vi "Asynchronous - Update RT to BC and RT to RT Data.vi"(5 "Raw Values (RT to BC)":T4, 7 "Map (RT to BC)":T1[](array[typedef]) {"Word Data Reference" format="%.0x"}, 8 "Error (in)":errorcluster, 9 "Updated FIFO Index []":i32[](array[numeric]), 10 "U16 []":u16[](array[numeric])) -> (0 "Error (out)":errorcluster)   [LabVIEW 2019, in "Ballard MIL-1553 Engine.lvlib"]
uses:
  Ballard MIL-1553 Engine.lvlib
  Controls/RT Async_Raw Values.ctl
  Controls/RT Async_Raw Values to Messages Index_Association.ctl
  Controls/RT Async_Map RT2BC.ctl
  <vilib>/NI VeriStand/Custom Device API/Data Reference.ctl
  Controls/RT Async_Map_Type.ctl
  <userlib>/_OpenG.lib/array/array.llb/Remove Duplicates from 1D Array (I32)__ogtk.vi
  <instrlib>/BTI1553Lib/BTI1553LV.lvlib
  <vilib>/NI VeriStand/Custom Device Tools/Custom Device Utility Library/Custom Device Utility Library.lvlib
  <vilib>/NI VeriStand/Custom Device API/Custom Device API.lvlib
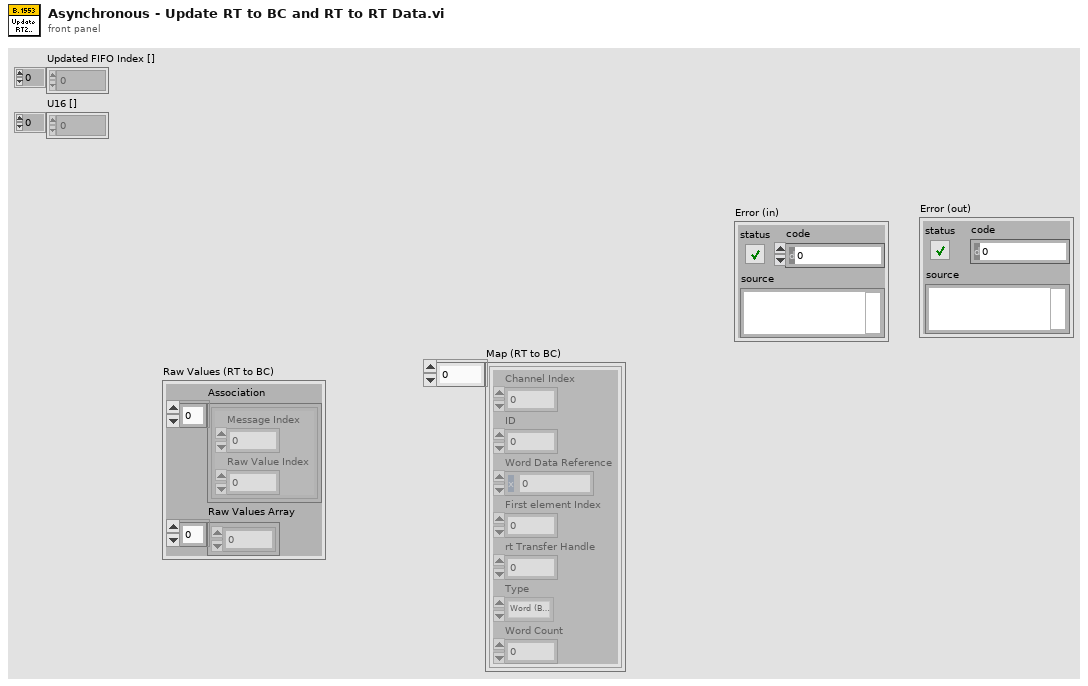
[diagram p1: front panel]
types:
  T1 = typedef "Ballard MIL-1553 Engine.lvlib/RT Async_Map RT2BC.ctl" = cluster{"Channel Index":i32, "ID":i32, "Word Data Reference":T2, "First element Index":i32, "rt Transfer Handle":u64, "Type":T3, "Word Count":i32}
  T2 = typedef "Custom Device API.lvlib/Data Reference.ctl" = i32
  T3 = typedef "Ballard MIL-1553 Engine.lvlib/RT Async_Map_Type.ctl" = enum16{"Word (BC to RT)", "Word (MC (Rx))", "Acyclic Message Trigger", "Word (RT to ..)", "Word (RT to RT)", "Word (MC (Tx))", "RT Status", "BC Commands", "RT Commands"}
  T4 = typedef "Ballard MIL-1553 Engine.lvlib/RT Async_Raw Values.ctl" = cluster{"Association":T5[], "Raw Values Array":u16[]}
  T5 = typedef "Ballard MIL-1553 Engine.lvlib/RT Async_Raw Values to Messages Index_Association.ctl" = cluster{"Message Index":i32, "Raw Value Index":i32}
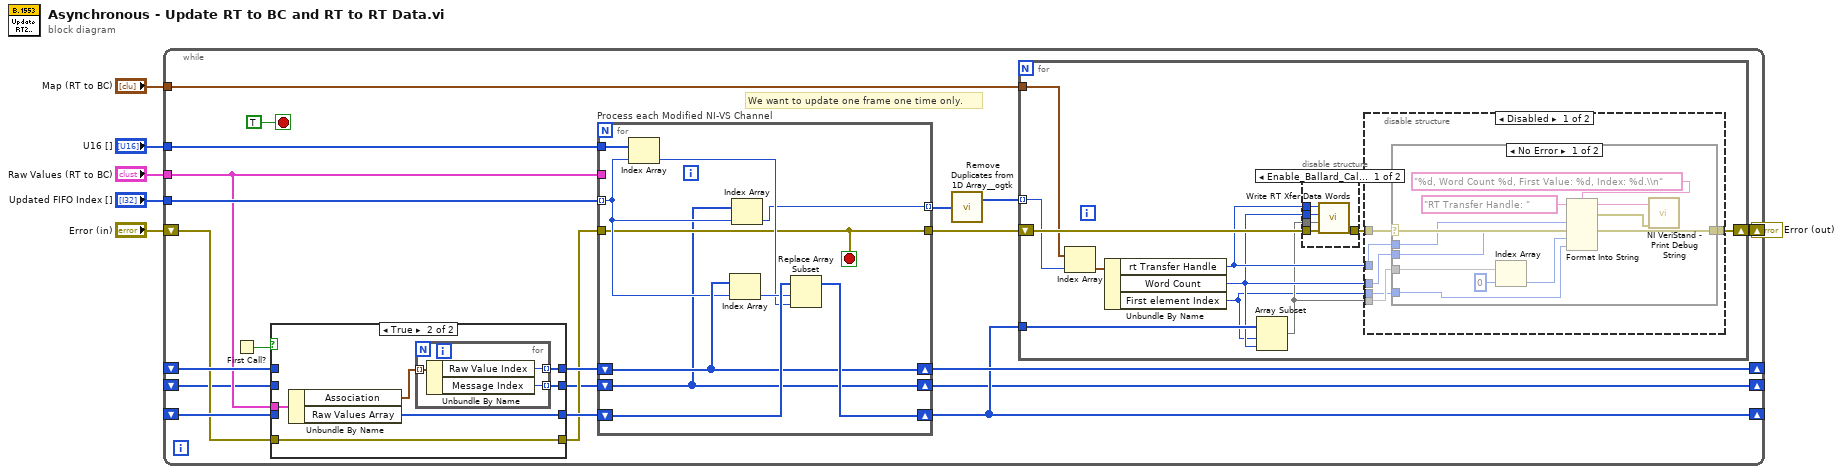
[diagram p0: block diagram]
diagram:
  n1 = while {
    tunnel: "Raw Values (RT to BC)" -> [w18]
    tunnel: "Updated FIFO Index []" -> [w27]
    tunnel: "U16 []" -> [w26]
    tunnel: "Map (RT to BC)" -> [w10]
    shift-right: [w14] -> w3
    shift-left: "Error (in)" -> [w17]
    shift-right: [w11] -> _
    shift-left: _ -> [w23]
    shift-right: [w21] -> _
    shift-left: _ -> [w20]
    shift-right: [w8] -> _
    shift-left: _ -> [w7]
    stop <- TRUE stop-if-true
    # "We want to update one frame one time only."
    n2 = First Call?() -> (First Call?: T/F=w19:bool)
    n3 = case shown="True" w19 {
      tunnel: w18 -> [_ w73]
      tunnel: [w67 w72] -> w24
      tunnel: w23 -> [w67 _]
      tunnel: [w66 w70] -> w22
      tunnel: w20 -> [w66 _]
      tunnel: w17 -> [w65 w69]
      tunnel: [w65 w69] -> w16
      tunnel: [w64 w68] -> w9
      tunnel: w7 -> [w64 _]
      frame False {
      }
      frame True {
        n4 = Unbundle By Name(w73) -> ("Association"=w71:T5[], "Raw Values Array"=w72:u16[])
        n5 = for {
          tunnel: w71 -> [w76] mode=indexing
          tunnel: [w75] -> w70 mode=indexing
          tunnel: [w74] -> w68 mode=indexing
          n6 = Unbundle By Name(w76) -> ("Raw Value Index"=w75:i32, "Message Index"=w74:i32)
        }
      }
    }
    n7 = for "Process each Modified NI-VS Channel" {
      tunnel: w18 -> [_]
      tunnel: w27 -> [w82] mode=indexing
      tunnel: w26 -> [w86]
      tunnel: w16 -> [w79]
      tunnel: [w79] -> w15
      shift-right: [w84] -> w11
      shift-left: w24 -> [w85]
      shift-right: [w83] -> w21
      shift-left: w22 -> [w83]
      tunnel: [w77] -> w13 mode=indexing
      shift-right: [w78] -> w8
      shift-left: w9 -> [w78]
      stop <- w79 stop-if-true
      n8 = Index Array(array=w86, index=w82) -> (element=w80:u16)
      n9 = Index Array(array=w83, index=w82) -> (element=w81:i32)
      n10 = Index Array(array=w78, index=w82) -> (element=w77:i32)
      n11 = Replace Array Subset(array=w85, new element=w80, index=w81) -> (w84:u16[])
    }
    n12 = call-poly <userlib>:"Remove Duplicates from 1D Array__ogtk.vi"("Input Array"=w13) -> ("Output Array"=w12:i32[])  [unwired: 1 out]
    n13 = for {
      shift-right: [w28] -> w14
      shift-left: w15 -> [w38]
      tunnel: w12 -> [w34] mode=indexing
      tunnel: w11 -> [w36]
      tunnel: w10 -> [w35]
      n14 = Index Array(array=w35, index=w34) -> (element=w37:T1)
      n15 = Unbundle By Name(w37) -> ("rt Transfer Handle"=w33:u64, "Word Count"=w32:i32, "First element Index"=w30:i32)
      n16 = Array Subset(array=w36, index=w30, length=w32) -> (w31:u16[])
      n17 = disable-structure shown="Enable_Ballard_Calls==True, Default" {
        disable-tunnel: w38 -> [w62 w63]
        disable-tunnel: [w61 w63] -> w29
        disable-tunnel: w33 -> [w60 _]
        disable-tunnel: w32 -> [w59 _]
        disable-tunnel: w31 -> [w58 _]
        frame condition #0 (active) {
          n18 = call <instrlib>:"Write RT Xfer Data Words.vi"("error in (no error)"=w62, "data words"=w58, "data word count in"=w59, "rt transfer handle in"=w60) -> ("error out"=w61:errorcluster)  [unwired: 5 in, 2 out]
        }
        frame condition #1 {
        }
      }
      n19 = disable-structure shown="Disabled" {
        disable-tunnel: w33 -> [w44 _]
        disable-tunnel: w32 -> [w43 _]
        disable-tunnel: w31 -> [w42 _]
        disable-tunnel: w30 -> [w41 _]
        disable-tunnel: w29 -> [w40 w57]
        disable-tunnel: [w39 w57] -> w28
        frame Disabled {
          n20 = case shown="No Error" w40 {
            selector: w40 -> [w55 w56]
            tunnel: [w55 w56] -> w39
            tunnel: w44 -> [w50 _]
            tunnel: w43 -> [w48 _]
            tunnel: w42 -> [w47 _]
            tunnel: w41 -> [w45 _]
            frame No Error {
              n21 = Index Array(array=w47, index=0) -> (element=w46:u16)
              n22 = Format Into String(format string="%d, Word Count %d, First Value: %d, Index: %d.\\n", initial string="RT Transfer Handle: ", w50, w48, w46, w45) -> (resulting string=w53:string, error out=w54:errorcluster)  [unwired: 1 in]
              n23 = call <vilib>:"NI VeriStand - Print Debug String.vi"("error in (no error)"=w54, "Message"=w53) -> ()  [unwired: 9 in, 1 out]
            }
            frame Error {
            }
          }
        }
        frame Enabled {
        }
      }
    }
  }
  "Error (out)" <- w3
